vi "emi_Get Sel ref if missing.vi"(5 "VI Refnum(Level)":refnum<vi>, 9 "error in (no error)":errorcluster, 13 "Level(This VI)":T1(ring)) -> (2 "Ref Generated":bool=TRUE, 6 "VI Refnum Out":refnum<vi>, 10 "error out":errorcluster)   [LabVIEW 2010]
doc: "If VI Refnum is connected to a valid ref number, nothing is done. If it is not, the ref number of the selected level caller is selected(This VI, Caller, Callers, caller)\n\nThe Idee: help making VIs that default to working with the VI they are placed on. \n\nOn Error In: No Action"
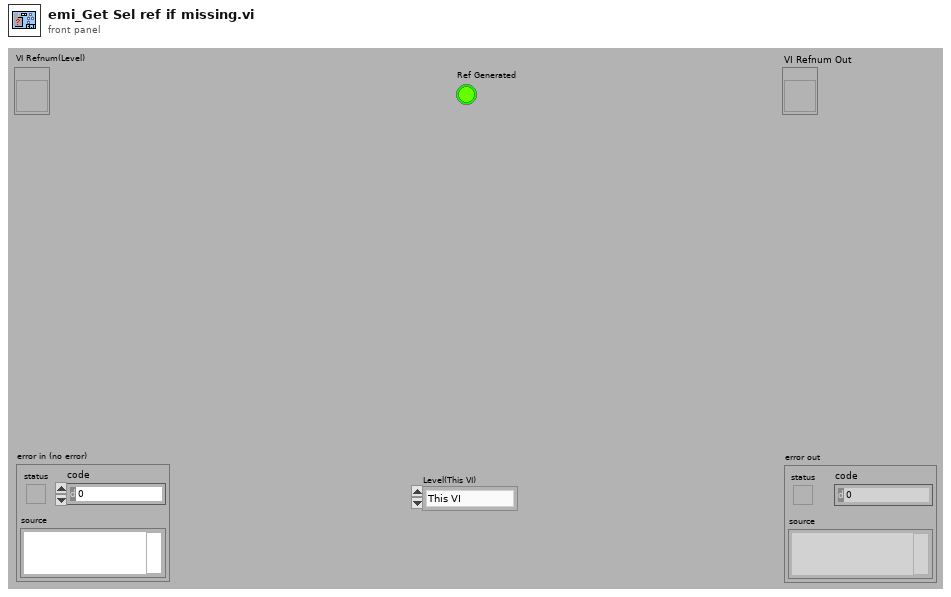
[diagram p1: front panel]
types:
  T1 = enum16{"This VI", "Caller(1)", "Caller's caller(2)", "Caller 3", "Caller 4", "Caller 5", "Caller 6", "Caller 7", "Caller 8", "Caller 9", "Caller 10", "Caller 11", "Caller 12"}
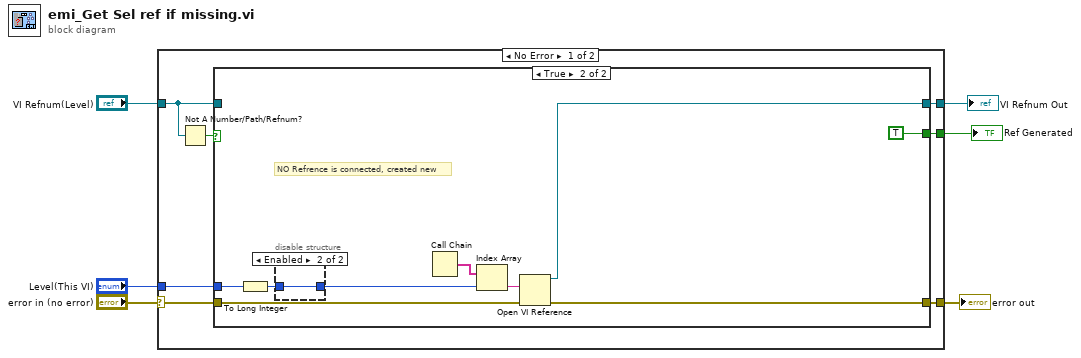
[diagram p0: block diagram]
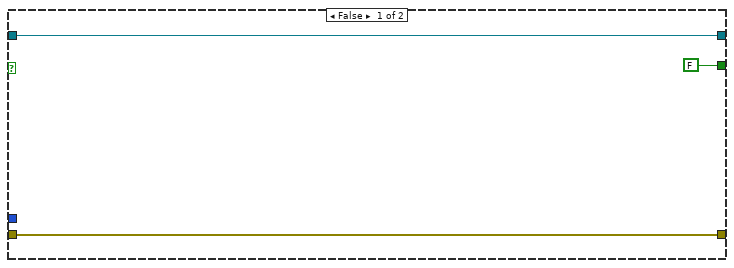
[diagram p2: hidden frame]
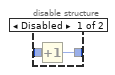
[diagram p3: hidden frame]
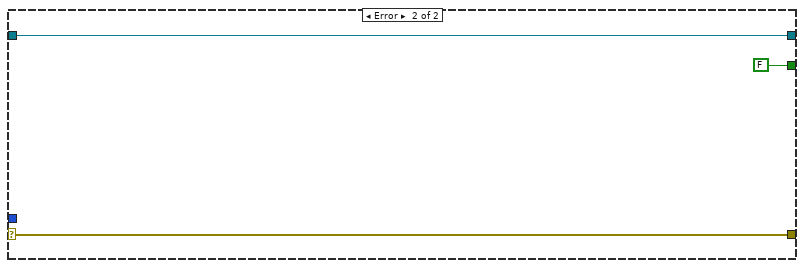
[diagram p4: hidden frame]
diagram:
  n1 = case shown="No Error" "error in (no error)" {
    selector: "error in (no error)" -> [w9 w31]
    tunnel: [w13 w31] -> w6
    tunnel: [w12 w30] -> w5
    tunnel: "VI Refnum(Level)" -> [w10 w30]
    tunnel: [w8 FALSE ("Ref Generated")] -> w2
    tunnel: "Level(This VI)" -> [w7 _]
    frame No Error {
      n2 = Not A Number/Path/Refnum?(number/path/refnum=w10) -> (NaN/Path/Refnum?=w11:bool)
      n3 = case shown="True" w11 {
        tunnel: [w15 w17] -> w13
        tunnel: [w16 w23] -> w12
        tunnel: w10 -> [w16 _]
        tunnel: w9 -> [w15 w21]
        tunnel: [FALSE ("Ref Generated") TRUE ("Ref Generated")] -> w8
        tunnel: w7 -> [_ w20]
        frame False {
        }
        frame True {
          # "NO Refrence is connected, created new"
          n4 = To Long Integer(number=w20) -> (32bit integer=w19:i32)
          n5 = disable-structure shown="Enabled" {
            disable-tunnel: w19 -> [w27 w28]
            disable-tunnel: [w26 w28] -> w18
            frame Disabled {
              n6 = Increment(x=w27) -> (x+1=w26:i32)
            }
            frame Enabled {
            }
          }
          n7 = Call Chain() -> (call chain=w25:string[])
          n8 = Index Array(array=w25, index=w18) -> (element=w24:string)
          n9 = Open VI Reference(vi path=w24, error in (no error)=w21) -> (vi reference=w23:refnum<vi>, error out=w17:errorcluster)  [unwired: 4 in]
        }
      }
    }
    frame Error {
    }
  }
  "error out" <- w6
  "Ref Generated" <- w2
  "VI Refnum Out" <- w5
